vi "Read Waveform Measurement.vi"(8 "error in (no error)":errorcluster {"code" format="%.0x"}, 9 "Measurement Function (Rise Time)":i32(ring) items=["Rise Time", "Fall Time", "Frequency", "Period", "Voltage RMS", "Voltage Vpp", "Voltage Max", "Voltage Min", "Voltage High", "Voltage Low", "Voltage Average", "Width Negative", "Width Positive", "Duty Cycle Negative", "Duty Cycle Positive", "Amplitude", "Voltage RMS (cycle)", "Voltage Average (cycle)", "Positive Overshoot", "Negative Overshoot", "Timing Burst Width"], 10 "Channel Name (Channel 1)":string(combo)="CH1", 11 "VISA Resource Name":refnum<visa-resource-name>) -> (0 "error out":errorcluster {"code" format="%.0x"}, 2 "Measurement":dbl format="%.2p", 3 "VISA Resource Name Out":refnum<visa-resource-name>)   [LabVIEW 2010, in "Tektronix TDS 3000 Series.lvlib"]
doc: "This VI obtains a waveform measurement and returns the measurement value. You specify a particular measurement type, such as rise time, frequency, and voltage peak-to-peak. The waveform on which the oscilloscope calculates the waveform measurement is from an acquisition that you previously initiated. \n\nUse the tktds3k Initiate Acquisition VI, tktds3k Read Waveform VI, or tktds3k Read Min Max Waveform VI to start an acquisition on the channels that you enable with the tktds3k Configure Channel VI. You call this VI separately for each waveform measurement you want to obtain on a specific channel.\n\nNotes:\n\n(1) You must configure the appropriate reference levels before you call this VI to take a rise time, fall time, width negative, width positive, duty cycle negative, or duty cycle positive measurement.\n\n(2) You configure the low, mid, and high references either by calling the Configure Reference Levels VI"
uses:
  <instrlib>/Tektronix TDS 3000 Series/Tektronix TDS 3000 Series.lvlib
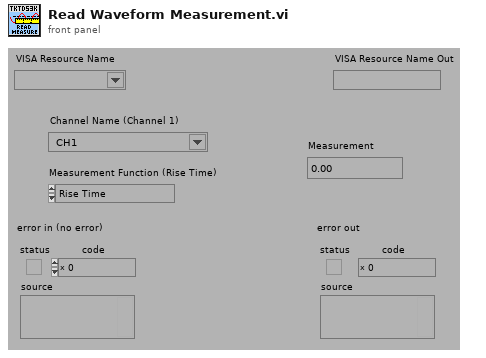
[diagram p1: front panel]
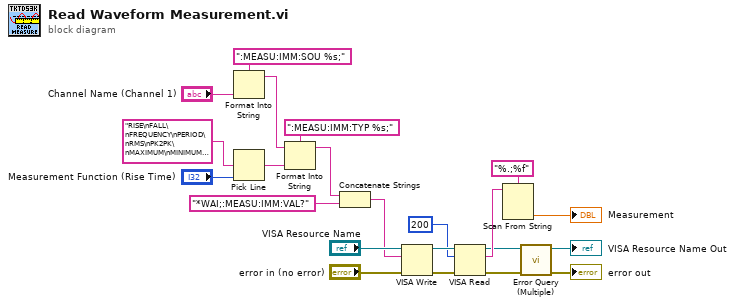
[diagram p0: block diagram]
diagram:
  n1 = Format Into String(format string=":MEASU:IMM:SOU %s;", "Channel Name (Channel 1)") -> (resulting string=w18:string)  [unwired: 2 in, 1 out]
  n2 = Pick Line(multi-line string="RISE\nFALL\nFREQUENCY\nPERIOD\nRMS\nPK2PK\nMAXIMUM\nMINIMUM\nHIGH\nLOW\nMEAN\nNWIDTH\nPWIDTH\nNDUTY\nPDUTY\nAMPLITUDE\nCRMS\nCMEAN\nPOVERSHOOT\nNOVERSHOOT\nBURST", line index="Measurement Function (Rise Time)") -> (output string=w19:string)  [unwired: 1 in]
  n3 = Format Into String(format string=":MEASU:IMM:TYP %s;", initial string=w18, w19) -> (resulting string=w10:string)  [unwired: 1 in, 1 out]
  n4 = Concatenate Strings(w10, "*WAI;:MEASU:IMM:VAL?" ("write buffer")) -> (w9:string)
  n5 = VISA Write(VISA resource name="VISA Resource Name", write buffer=w9, error in (no error)="error in (no error)") -> (VISA resource name out=w13:refnum<visa-resource-name>, error out=w12:errorcluster)  [unwired: 1 out]
  n6 = VISA Read(VISA resource name=w13, byte count=u32 200, error in (no error)=w12) -> (VISA resource name out=w2:refnum<visa-resource-name>, read buffer=w6:string, error out=w4:errorcluster)  [unwired: 1 out]
  n7 = Scan From String(format string="%.;%f", input string=w6) -> (output 1=→"Measurement":dbl)  [unwired: 3 in, 3 out]
  n8 = call <instrlib>:"Error Query (Multiple).vi"("error in (no error)"=w4, "VISA Resource Name"=w2) -> ("error out"=→"error out":errorcluster, "VISA Resource Name Out"=→"VISA Resource Name Out":refnum<visa-resource-name>)  [unwired: 6 in, 2 out]
